vi "Text 2 Source Group.vi"(10 "Text":string) -> (2 "Source Group":T1)   [LabVIEW 2013]
uses:
  Names/Source Group Type.ctl
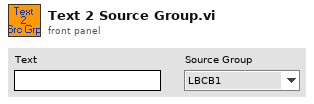
[diagram p1: front panel]
types:
  T1 = typedef "Source Group Type.ctl" = enum16{"LBCB1", "LBCB2", "Consolidated", "External"}
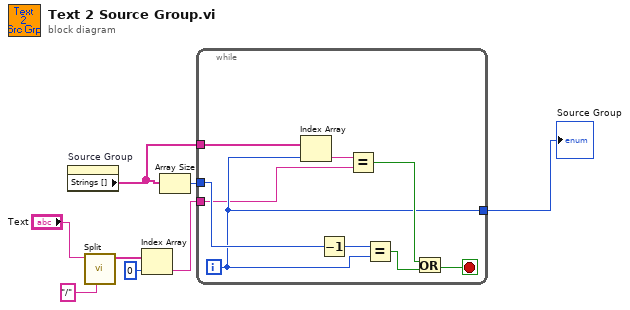
[diagram p0: block diagram]
diagram:
  n1 = property on="Source Group" class="Enum (strict)"() -> ("Strings []"=w7:string[])  [unwired: 2 in, 2 out]
  n2 = call "Split.vi"("delimiter"="/", "String"="Text") -> ("Array Result"=w4:string[])  [unwired: 9 in]
  n3 = Index Array(array=w4, index=0) -> (element=w1:string)
  n4 = Array Size(array=w7) -> (size(s)=w6:i32)
  n5 = while {
    tunnel: w7 -> [w17]
    tunnel: w1 -> [w9]
    tunnel: [w11] -> w8
    tunnel: w6 -> [w15]
    i -> [w11]
    stop <- w13 stop-if-true
    n6 = Index Array(array=w17, index=w11) -> (element=w10:string)
    n7 = Decrement(x=w15) -> (x-1=w14:i32)
    n8 = Equal?(x=w10, y=w9) -> (x = y?=w16:bool)
    n9 = Equal?(x=w14, y=w11) -> (x = y?=w12:bool)
    n10 = Or(x=w16, y=w12) -> (x .or. y?=w13:bool)
  }
  "Source Group" <- w8
